vi "Read Power Meter Data.vi"(0 "VISA resource name":refnum<visa-resource-name>, 5 "Unit (0:dBm)":i32(ring) items=["dBm", "Watt", "dB"], 11 "error in (no error)":errorcluster) -> (4 "VISA resource name out":refnum<visa-resource-name>, 6 "Power Measurement":dbl, 8 "Measurement Status":i32, 10 "Power Sensor Connection":i32(ring) items=["Not Connected", "Connected"], 14 "Port Number":i32, 15 "error out":errorcluster)   [LabVIEW 2020, in "Anritsu Signal Analyzer Series.lvlib"]
doc: "Reads the power and Power Meter status."
uses:
  Anritsu Signal Analyzer Series.lvlib
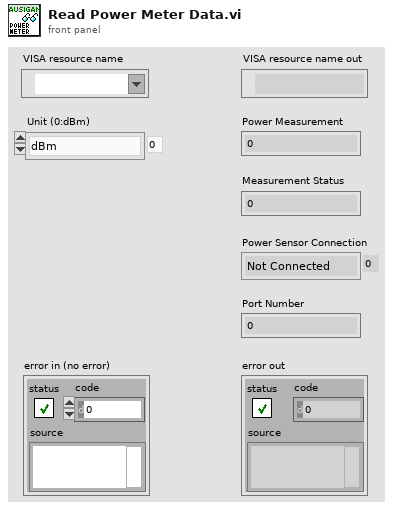
[diagram p1: front panel]
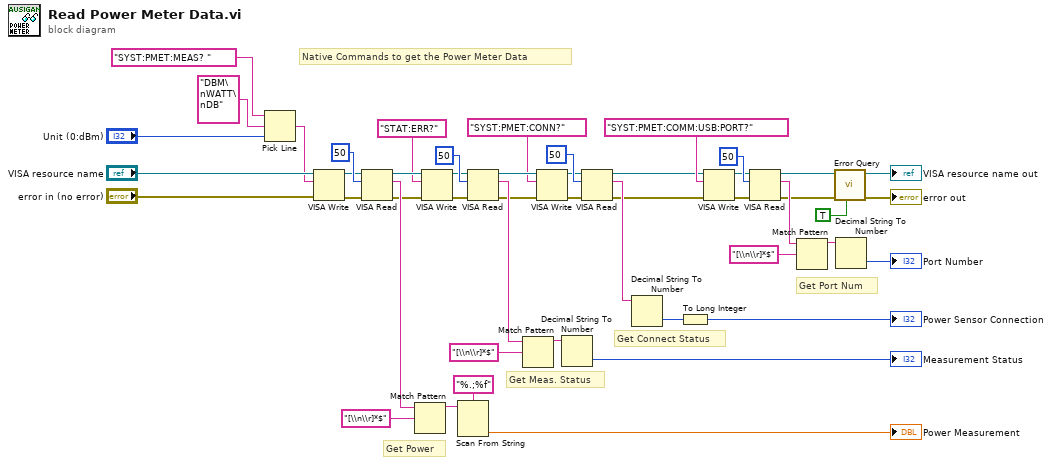
[diagram p0: block diagram]
diagram:
  # "Native Commands to get the Power Meter Data"
  # "Get Port Num"
  # "Get Connect Status"
  # "Get Meas. Status"
  # "Get Power"
  n1 = Pick Line(string ("")="SYST:PMET:MEAS? " ("_CommandGet"), multi-line string="DBM\nWATT\nDB", line index="Unit (0:dBm)") -> (output string=w6:string)
  n2 = VISA Write(VISA resource name="VISA resource name", write buffer=w6, error in (no error)="error in (no error)") -> (VISA resource name out=w37:refnum<visa-resource-name>, error out=w38:errorcluster)  [unwired: 1 out]
  n3 = VISA Read(VISA resource name=w37, byte count=u32 50 ("byte count (0)"), error in (no error)=w38) -> (VISA resource name out=w31:refnum<visa-resource-name>, read buffer=w41:string, error out=w30:errorcluster)  [unwired: 1 out]
  n4 = Match Pattern(string=w41, regular expression="[\\n\\r]*$") -> (before substring=w10:string)  [unwired: 1 in, 3 out]
  n5 = VISA Write(VISA resource name=w31, write buffer="STAT:ERR?" ("_CommandGet"), error in (no error)=w30) -> (VISA resource name out=w32:refnum<visa-resource-name>, error out=w29:errorcluster)  [unwired: 1 out]
  n6 = Scan From String(format string="%.;%f" ("形式文字列"), input string=w10) -> (output 1=→"Power Measurement":dbl)  [unwired: 3 in, 3 out]
  n7 = VISA Read(VISA resource name=w32, byte count=u32 50 ("byte count (0)"), error in (no error)=w29) -> (VISA resource name out=w24:refnum<visa-resource-name>, read buffer=w35:string, error out=w23:errorcluster)  [unwired: 1 out]
  n8 = Match Pattern(string=w35, regular expression="[\\n\\r]*$") -> (before substring=w36:string)  [unwired: 1 in, 3 out]
  n9 = VISA Write(VISA resource name=w24, write buffer="SYST:PMET:CONN?", error in (no error)=w23) -> (VISA resource name out=w26:refnum<visa-resource-name>, error out=w25:errorcluster)  [unwired: 1 out]
  n10 = Decimal String To Number(string=w36) -> (number=→"Measurement Status":i32)  [unwired: 2 in, 1 out]
  n11 = VISA Read(VISA resource name=w26, byte count=u32 50 ("バイトカウント"), error in (no error)=w25) -> (VISA resource name out=w3:refnum<visa-resource-name>, read buffer=w28:string, error out=w2:errorcluster)  [unwired: 1 out]
  n12 = Decimal String To Number(string=w28) -> (number=w22:i32)  [unwired: 2 in, 1 out]
  n13 = To Long Integer(number=w22) -> (32bit integer=→"Power Sensor Connection":i32)
  n14 = VISA Write(VISA resource name=w3, write buffer="SYST:PMET:COMM:USB:PORT?" ("_CommandGet"), error in (no error)=w2) -> (VISA resource name out=w16:refnum<visa-resource-name>, error out=w17:errorcluster)  [unwired: 1 out]
  n15 = VISA Read(VISA resource name=w16, byte count=u32 50 ("byte count (0)"), error in (no error)=w17) -> (VISA resource name out=w14:refnum<visa-resource-name>, read buffer=w20:string, error out=w15:errorcluster)  [unwired: 1 out]
  n16 = Match Pattern(string=w20, regular expression="[\\n\\r]*$") -> (before substring=w21:string)  [unwired: 1 in, 3 out]
  n17 = call "Error Query.vi"("Enable Power Meter Error (F:Disable)"=TRUE, "error in (no error)"=w15, "VISA resource name"=w14) -> ("error out"=→"error out":errorcluster, "VISA resource name out"=→"VISA resource name out":refnum<visa-resource-name>)  [unwired: 5 in, 2 out]
  n18 = Decimal String To Number(string=w21) -> (number=→"Port Number":i32)  [unwired: 2 in, 1 out]
